vi "Write secondsArc.vi"(8 "error in (no error)":errorcluster, 10 "secondsArc":dbl[unit] min=0.0 max=0.0002908882086657216, 11 "Elevation in":refnum<class "Elevation.lvclass">) -> (0 "error out":errorcluster, 3 "Elevation out":refnum<class "Elevation.lvclass">)   [LabVIEW 2022 SP3, in "TCSDataDefinitions.lvlib" / "TCSCommand.lvlib" / "TargetConfiguration.lvlib" / "Target.lvlib" / "FixedTarget.lvlib" / "Elevation.lvclass"]
uses:
  Elevation.lvclass
  Elevation.lvclass/Elevation.ctl
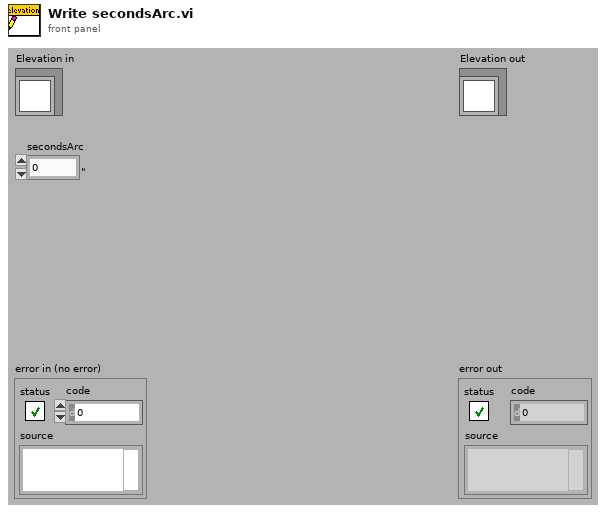
[diagram p1: front panel]
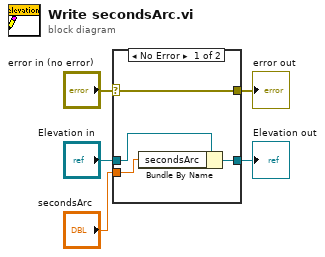
[diagram p0: block diagram]
diagram:
  n1 = case shown="No Error" "error in (no error)" {
    selector: "error in (no error)" -> [w9 w10]
    tunnel: [w9 w10] -> w4
    tunnel: [w7 w11] -> w2
    tunnel: "Elevation in" -> [w8 w11]
    tunnel: "secondsArc" -> [w6 _]
    frame No Error {
      n2 = Bundle By Name(cluster=w8, "secondsArc"=w6) -> (w7:refnum<class "Elevation.lvclass">)
    }
    frame Error {
    }
  }
  "error out" <- w4
  "Elevation out" <- w2
